vi "SetAllowedViInfomation.vi"(8 "error in (no error)":errorcluster caption="错误输入（无错误）", 11 "PanelExample 输入":refnum<class "PanelExample.lvclass"> caption="DNL_LabVIEW Object in") -> (0 "error out":errorcluster caption="错误输出", 1 "ViPath":path[](array[path]), 2 "ViAlias":string[](array[string]), 3 "PanelExample 输出":refnum<class "PanelExample.lvclass"> caption="DNL_LabVIEW Object out")   [LabVIEW 2013, in "PanelExample.lvclass"]
uses:
  PanelExample.lvclass
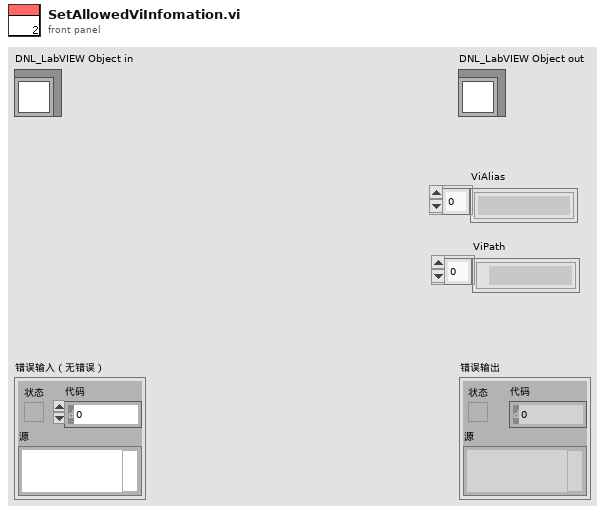
[diagram p1: front panel]
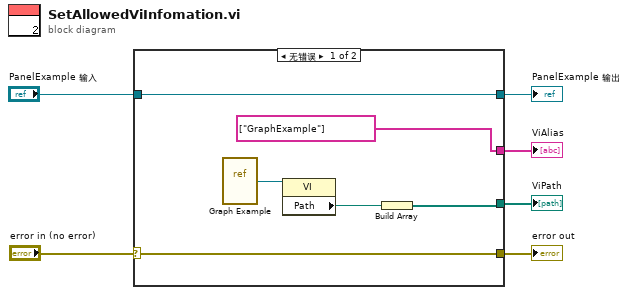
[diagram p0: block diagram]
diagram:
  n1 = case shown="无错误" "error in (no error)" {
    selector: "error in (no error)" -> [w12 w13]
    tunnel: [w12 w13] -> w5
    tunnel: "PanelExample 输入" -> [w11 w14]
    tunnel: [w11 w14] -> w3
    tunnel: [string[] ["GraphExample"] _] -> w2
    tunnel: [w8 _] -> w1
    frame No Error {
      n2 = vi-ref "Graph Example.vi"() -> (w10:refnum<vi>)
      n3 = property class="VI"(reference=w10) -> ("Path"=w9:path)  [unwired: 1 in, 2 out]
      n4 = Build Array(w9) -> (w8:path[])
    }
    frame Error {
    }
  }
  "error out" <- w5
  "PanelExample 输出" <- w3
  "ViAlias" <- w2
  "ViPath" <- w1
